vi "Close.vi"(8 "error in (no error)":errorcluster, 11 "LiDAR in":refnum<class "Telnet V2.lvclass">) -> (0 "error out":errorcluster)   [LabVIEW 2018, in "Telnet V2.lvlib" / "Telnet V2.lvclass"]
uses:
  Telnet V2.lvclass
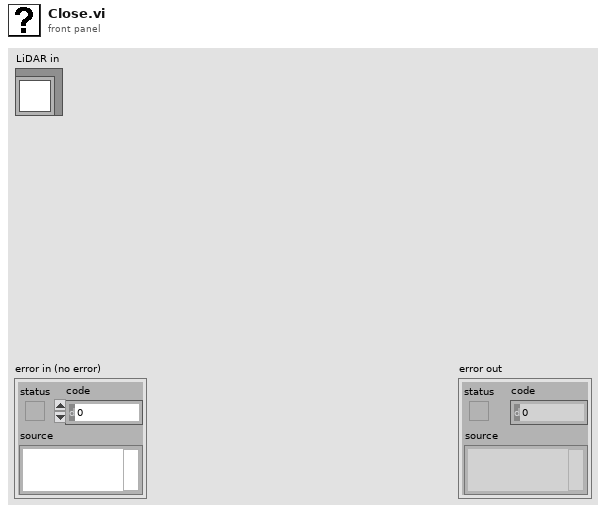
[diagram p1: front panel]
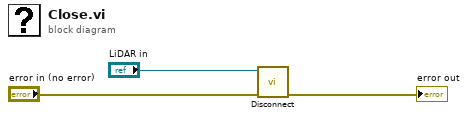
[diagram p0: block diagram]
diagram:
  n1 = call-dynamic "Disconnect.vi"("error in (no error)"="error in (no error)", "LiDAR in"="LiDAR in") -> ("error out"=→"error out":errorcluster)  [unwired: 8 in, 1 out]
